vi "VI Schedule Seite.vi"() -> ()   [LabVIEW 2020, in "Schedule Modul.lvlib"]
uses:
  Schedule Modul.lvlib
  Aktive Wochentage.ctl
  Zeitstempel.ctl
  Zeitstempel-Bedienelement.ctl
  Testreihenfolge.ctl
  Test-Auswahlfeld.ctl
  Planer Status.ctl
  Ergebnis Tabelle.ctl
  Aktion FGV Schedule Daten.ctl
  Aktion FGV Schedule Log.ctl
  Sprachverwaltung/Sprachverwaltung.lvlib
panel:
  in  "Testreihenfolge AK":T1 caption="Reihenfolge:" {"Test 5" items=[" ---", "Dichtheitstest", "Kalibrieren", "Cal-Gas Test", "T90 Test"]; "Test 4" items=[" ---", "Dichtheitstest", "Kalibrieren", "Cal-Gas Test", "T90 Test"]; "Test 3" items=[" ---", "Dichtheitstest", "Kalibrieren", "Cal-Gas Test", "T90 Test"]; "Test 2" items=[" ---", "Dichtheitstest", "Kalibrieren", "Cal-Gas Test", "T90 Test"]; "Test 1" items=[" ---", "Dichtheitstest", "Kalibrieren", "Cal-Gas Test", "T90 Test"]}
  out "Ergebnisse":T3
  in  "Auto Scheduler Status:":T4 caption="Ring" items=["inaktiv", "aktiv"]
  in  "Testreihenfolge:":T1 caption="Reihenfolge:" {"Test 5" items=[" ---", "Dichtheitstest", "Kalibrieren", "Cal-Gas Test", "T90 Test"]; "Test 4" items=[" ---", "Dichtheitstest", "Kalibrieren", "Cal-Gas Test", "T90 Test"]; "Test 3" items=[" ---", "Dichtheitstest", "Kalibrieren", "Cal-Gas Test", "T90 Test"]; "Test 2" items=[" ---", "Dichtheitstest", "Kalibrieren", "Cal-Gas Test", "T90 Test"]; "Test 1" items=[" ---", "Dichtheitstest", "Kalibrieren", "Cal-Gas Test", "T90 Test"]}
  in  "Zeiten":T5 {"Sonntag" format="%<%H:%M>T"; "Samstag" format="%<%H:%M>T"; "Freitag" format="%<%H:%M>T"; "Donnerstag" format="%<%H:%M>T"; "Mittwoch" format="%<%H:%M>T"; "Dienstag" format="%<%H:%M>T"; "Montag" format="%<%H:%M>T"}
  in  "Aktive Wochentage":T7
  # "Scheduler"
  # "Zeitgesteuerte Routine"
  # "Manuelle/Remote Routine"
  # "Ergebnisse"
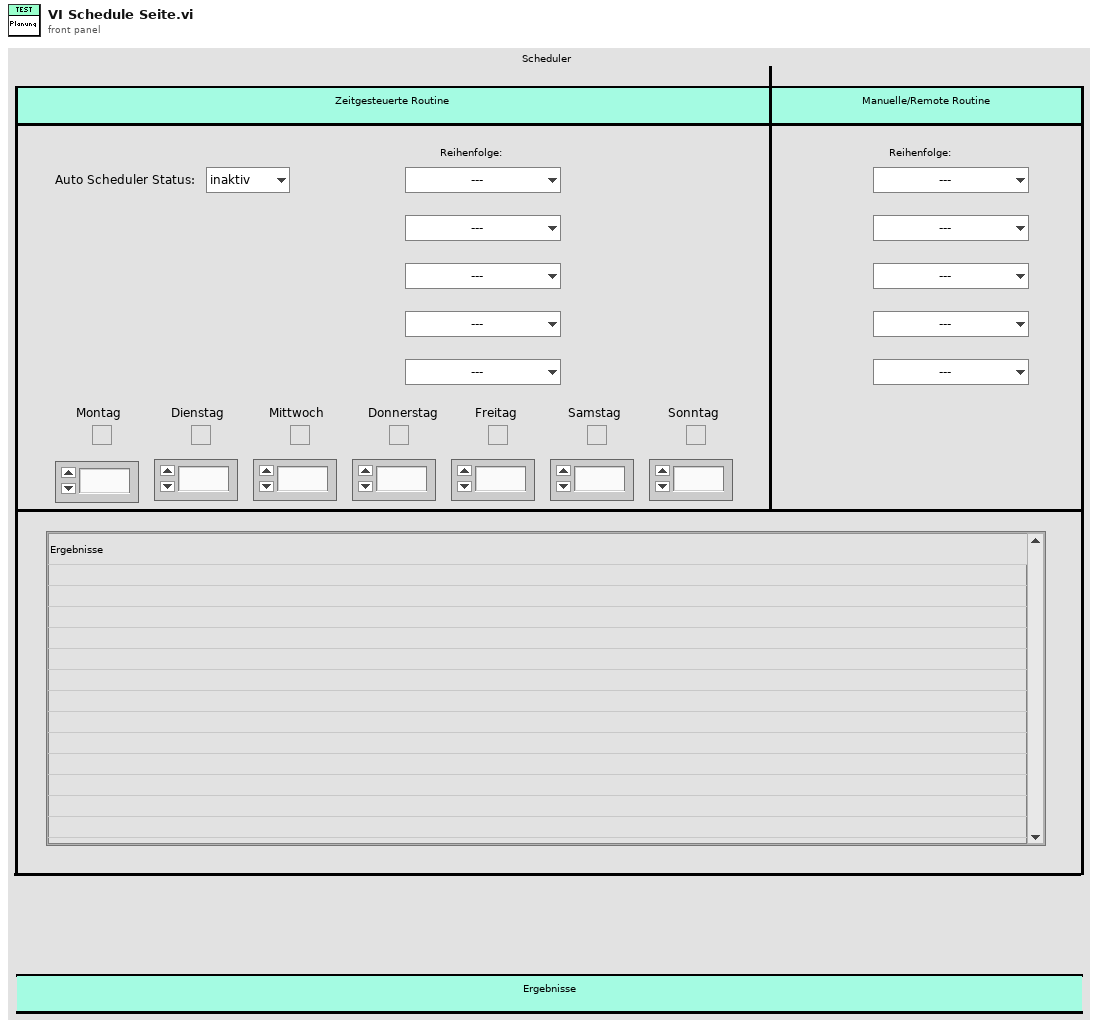
[diagram p1: front panel]
types:
  T1 = typedef "Schedule Modul.lvlib/Testreihenfolge.ctl" = cluster{"Test 1":T2, "Test 2":T2, "Test 3":T2, "Test 4":T2, "Test 5":T2}
  T2 = typedef "Schedule Modul.lvlib/Test-Auswahlfeld.ctl" = u16
  T3 = typedef "Schedule Modul.lvlib/Ergebnis Tabelle.ctl" = string[][]
  T4 = typedef "Schedule Modul.lvlib/Planer Status.ctl" = u16
  T5 = typedef "Schedule Modul.lvlib/Zeitstempel.ctl" = cluster{"Montag":T6, "Dienstag":T6, "Mittwoch":T6, "Donnerstag":T6, "Freitag":T6, "Samstag":T6, "Sonntag":T6}
  T6 = typedef "Schedule Modul.lvlib/Zeitstempel-Bedienelement.ctl" = timestamp
  T7 = typedef "Schedule Modul.lvlib/Aktive Wochentage.ctl" = cluster{"Montag":bool, "Dienstag":bool, "Mittwoch":bool, "Donnerstag":bool, "Freitag":bool, "Samstag":bool, "Sonntag":bool}
  T8 = typedef "Schedule Modul.lvlib/Aktion FGV Schedule Log.ctl" = enum16{"lesen", "neuer Eintrag", "laden", "löschen", "Anzeige löschen"}
  T9 = typedef "Schedule Modul.lvlib/Aktion FGV Schedule Daten.ctl" = enum16{"lesen", "laden", "speichern", "schreiben"}
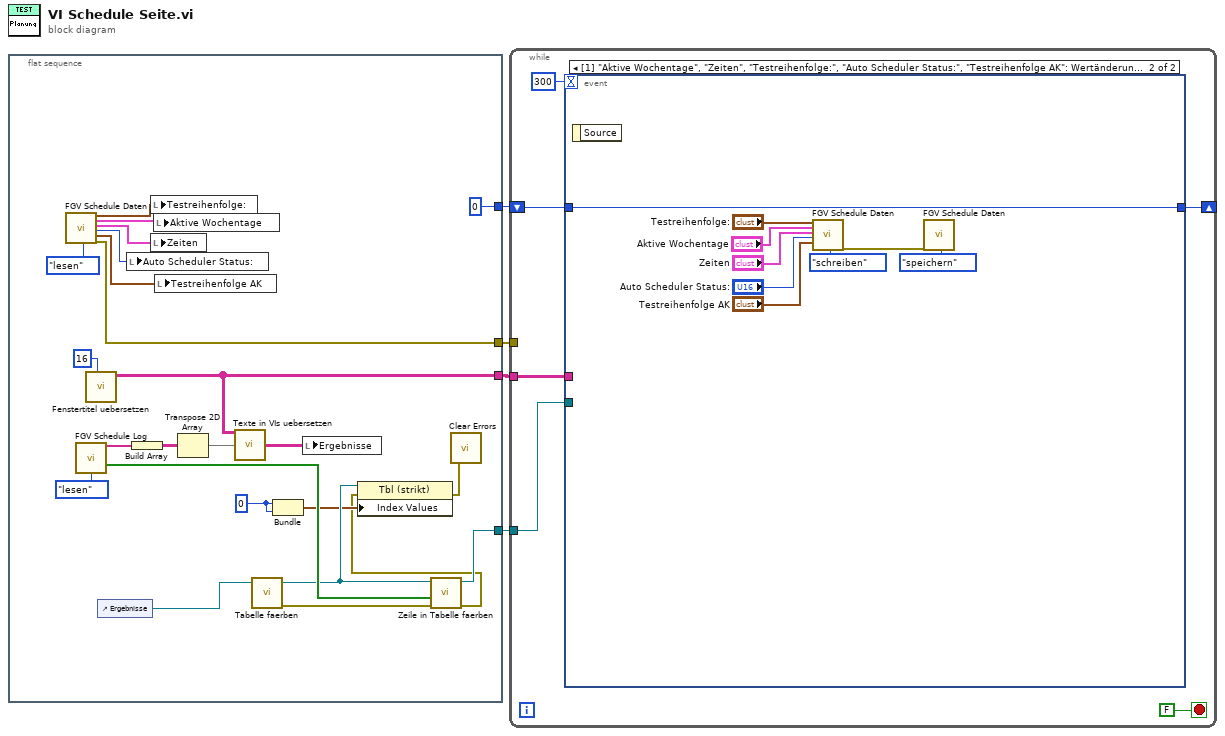
[diagram p0: block diagram]
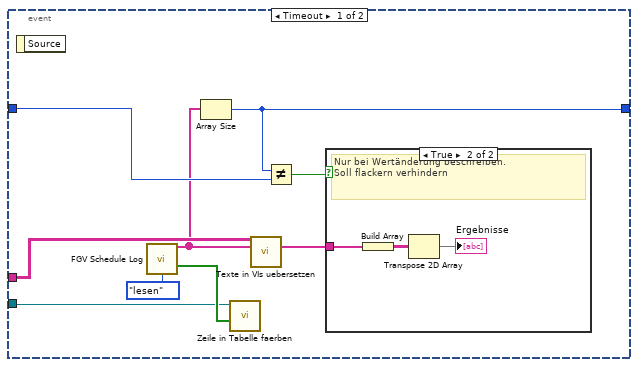
[diagram p2: hidden frame]
diagram:
  n1 = flat-sequence {
    tunnel: [w23] -> w4
    tunnel: [w14] -> w3
    tunnel: [0] -> w2
    tunnel: [w5] -> w1
    frame #0 {
      w9 = u32 0 ("Column")
      n2 = call "FGV Schedule Daten.vi"("Aktion"=Aktion_FGV_Schedule_Daten."lesen") -> ("Testreihenfolge:"=w25:T1, "Aktive Wochentage"=w22:T7, "Zeiten"=w24:T5, "Planer Status"=w18:T4, "Testreihenfolge AK"=w17:T1, "error out"=w23:errorcluster)  [unwired: 13 in]
      n3 = call "FGV Schedule Log.vi"("Aktion"=Aktion_FGV_Schedule_Log."lesen") -> ("Anzeige"=w20:string[], "Fehler"=w15:bool[])  [unwired: 11 in, 2 out]
      n4 = call "Fenstertitel uebersetzen.vi"("Index (Seite)"=16) -> ("Sprachliste"=w5:string[][])  [unwired: 7 in, 3 out]
      n5 = control-ref of="Ergebnisse"() -> (w14:refnum<vi>)
      n6 = local write "Auto Scheduler Status:"(w18) -> ()
      n7 = Build Array(w20) -> (w19:string[][])
      n8 = local write "Testreihenfolge:"(w25) -> ()
      n9 = local write "Zeiten"(w24) -> ()
      n10 = local write "Aktive Wochentage"(w22) -> ()
      n11 = local write "Testreihenfolge AK"(w17) -> ()
      n12 = Transpose 2D Array(2D array=w19) -> (transposed array=w6:string[][])
      n13 = call "Texte in VIs uebersetzen.vi"("Sprachliste"=w5, "2D String-Array zum Übersetzen"=w6) -> ("2D String-Array zum Übersetzen"=w7:string[][])  [unwired: 9 in, 4 out]
      n14 = call "Tabelle faerben.vi"("Ergebnisse"=w14) -> ("error out"=w16:errorcluster)  [unwired: 10 in]
      n15 = Bundle("Column"=w9, "Column"=w9) -> (w13:cluster{"Column":u32, "Column":u32})  [unwired: 1 in]
      n16 = local write "Ergebnisse"(w7) -> ()
      n17 = call "Zeile in Tabelle faerben.vi"("error in (no error)"=w16, "Fehler"=w15, "Ergebnisse"=w14) -> ("error out"=w12:errorcluster)  [unwired: 8 in]
      n18 = property class="Tbl (strikt)"(reference=w14, error in=w12, "Index Values"=w13) -> (error out=w11:errorcluster)  [unwired: 1 out]
      n19 = call <vilib>:"Clear Errors.vi"("error in (no error)"=w11) -> ()  [unwired: 5 in, 2 out]
    }
  }
  n20 = while {
    tunnel: w4 -> [_]
    tunnel: w3 -> [w30]
    shift-right: [w29] -> _
    shift-left: w2 -> [w28]
    tunnel: w1 -> [w27]
    stop <- FALSE stop-if-true
    n21 = event shown="[1] \"Aktive Wochentage\", \"Zeiten\", \"Testreihenfolge:\", \"Auto Scheduler Status:\", \"Testreihenfolge AK\": Wertänderung" {
      selector: _ -> [_ _]
      dyn-events: _ -> [_ _]
      timeout: 300 -> [_ _]
      tunnel: w30 -> [w39 _]
      tunnel: [w37 w45] -> w29
      tunnel: w28 -> [w36 w45]
      tunnel: w27 -> [w35 _]
      event Timeout {
        n22 = event-data() -> ()  [unwired: 1 in, 1 out]
        n23 = call "FGV Schedule Log.vi"("Aktion"=Aktion_FGV_Schedule_Log."lesen") -> ("Anzeige"=w34:string[], "Fehler"=w40:bool[])  [unwired: 11 in, 2 out]
        n24 = Array Size(array=w34) -> (size(s)=w37:i32)
        n25 = call "Zeile in Tabelle faerben.vi"("Fehler"=w40, "Ergebnisse"=w39) -> ()  [unwired: 9 in, 1 out]
        n26 = call "Texte in VIs uebersetzen.vi"("Sprachliste"=w35, "String-Array zum Übersetzen"=w34) -> ("String-Array zum Übersetzen"=w33:string[])  [unwired: 9 in, 4 out]
        n27 = Not Equal?(x=w37, y=w36) -> (x != y?=w38:bool)
        n28 = case shown="True" w38 {
          tunnel: w33 -> [_ w42]
          frame False {
          }
          frame True {
            # "Nur bei Wertänderung beschreiben.\nSoll flackern verhindern"
            n29 = Build Array(w42) -> (w44:string[][])
            n30 = Transpose 2D Array(2D array=w44) -> (transposed array=→"Ergebnisse":string[][])
          }
        }
      }
      event Value Change {
        n31 = event-data() -> ()  [unwired: 1 in, 1 out]
        n32 = call "FGV Schedule Daten.vi"("Testreihenfolge:"="Testreihenfolge:", "Aktive Wochentage"="Aktive Wochentage", "Zeiten"="Zeiten", "Planer Status"="Auto Scheduler Status:", "Testreihenfolge AK"="Testreihenfolge AK", "Aktion"=Aktion_FGV_Schedule_Daten."schreiben") -> ("error out"=w48:errorcluster)  [unwired: 8 in, 5 out]
        n33 = call "FGV Schedule Daten.vi"("error in (no error)"=w48, "Aktion"=Aktion_FGV_Schedule_Daten."speichern") -> ()  [unwired: 12 in, 6 out]
      }
    }
  }
